vi "Carbide-Open.vi"(10 "Laser IP address":string) -> (0 "Error Out":errorcluster)   [LabVIEW 2014]
doc: "André Romero - 2021\nandretec@ifsc.usp.br\nIFSC - USP"
uses:
  <vilib>/httpClient/ClientHandle.ctl
  Carbide-Global.vi
  <vilib>/httpClient/LabVIEWHTTPClient.lvlib
panel:
  out "body":string
  out "Refnum out":T1
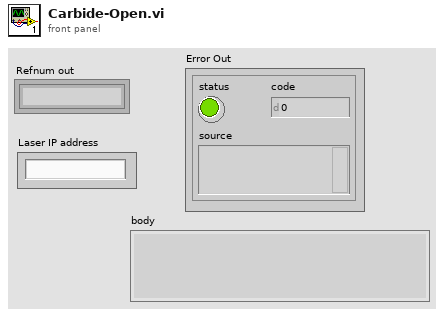
[diagram p1: front panel]
types:
  T1 = typedef "LabVIEWHTTPClient.lvlib/ClientHandle.ctl" = refnum<k1>
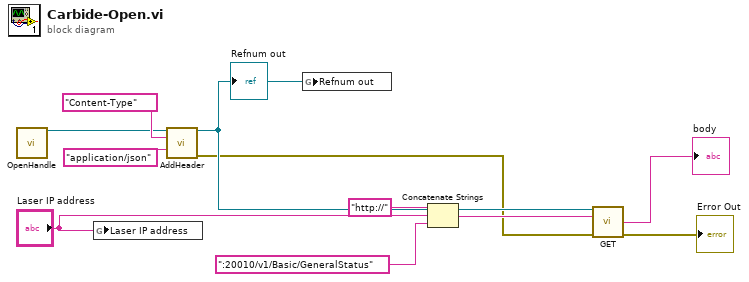
[diagram p0: block diagram]
diagram:
  n1 = call <vilib>:"OpenHandle.vi"() -> ("client handle out"=w9:T1)  [unwired: 14 in, 1 out]
  n2 = global write "Carbide-Global.vi" "Laser IP address"("Laser IP address") -> ()
  n3 = call <vilib>:"AddHeader.vi"("client handle"=w9, "header"="Content-Type", "value"="application/json") -> ("client handle out"=w5:T1, "error out"=w2:errorcluster)  [unwired: 11 in]
  "Refnum out" <- w5
  n4 = global write "Carbide-Global.vi" "Refnum out"(w5) -> ()
  n5 = Concatenate Strings("http://" ("string"), "Laser IP address", ":20010/v1/Basic/GeneralStatus" ("string")) -> (w8:string)
  n6 = call <vilib>:"GET.vi"("client handle"=w5, "url"=w8, "error in (no error)"=w2) -> ("body"=→"body":string, "error out"=→"Error Out":errorcluster)  [unwired: 9 in, 2 out]
